vi "gfitsio-read-key-logical.vi"(7 "keyname":string, 8 "error in (no error)":errorcluster, 9 "default value":bool, 11 "gfits refnum":T1) -> (0 "error out":errorcluster, 1 "comment":string, 2 "value":bool, 3 "dup gfits refnum":T1)   [LabVIEW 2022 SP3, in "gfitsio.lvlib"]
doc: "Return the specified keyword. <B>default value</B> specifies the desired returned data type of the keyword value. Data type conversion will be performed for numeric values if the keyword value does not have the same data type. If the keyword does not exist or an error occurs <B>value</B> will be equal to <B>default value</B>."
uses:
  gfitsio.lvlib
  gfitsio-refnum.ctl
  cfitsio-datatypes.ctl
  gfitsio.dll
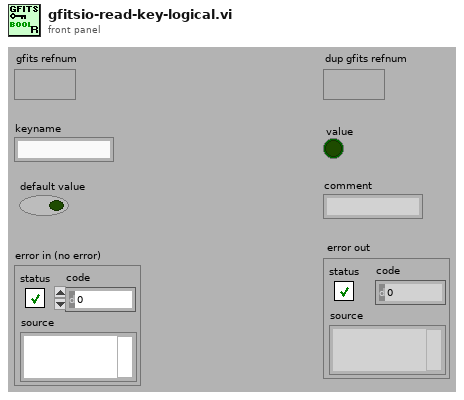
[diagram p1: front panel]
types:
  T1 = typedef "gfitsio.lvlib/gfitsio-refnum.ctl" = refnum<k1>
  T2 = typedef "gfitsio.lvlib/cfitsio-datatypes.ctl" = i32
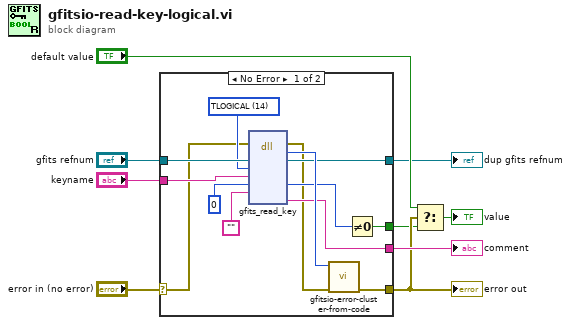
[diagram p0: block diagram]
diagram:
  n1 = case shown="No Error" "error in (no error)" {
    selector: "error in (no error)" -> [w11 w24]
    tunnel: [w21 w24] -> w3
    tunnel: "gfits refnum" -> [w19 w23]
    tunnel: [w20 w23] -> w1
    tunnel: "keyname" -> [w17 _]
    tunnel: [w12 _] -> w2
    tunnel: [w14 _] -> w4
    frame No Error {
      w18 = T2 14 items=["TBIT"=1, "TBYTE  (U8)"=11, "TSBYTE  (I8)"=12, "TLOGICAL"=14, "TSTRING"=16, "TUSHORT  (U16)"=20, "TSHORT  (I16)"=21, "TUINT"=31, "TULONG  (U32)"=40, "TLONG  (I32)"=41, "TFLOAT  (SGL)"=42, "TLONGLONG  (I64)"=81, "TDOUBLE  (DBL)"=82, "TCOMPLEX  (CSG)"=83, "TDOUBLECOMPLEX  (CDB)"=163] ("cfitsio datatype")
      n2 = dll-call lib="gfitsio.dll" fn="gfits_read_key"(error in=w11, "gfits refnum"=w19, "datatype"=w18, "keyname"=w17, "value"=u8 0, "units"="") -> (error out=w10:errorcluster, w22:i32, "gfits refnum"=w20:T1, "value"=w15:u8, "comment"=w14:string)  [unwired: 4 in, 3 out]
      n3 = call "gfitsio-error-cluster-from-code.vi"("error in (no error)"=w10, "error code"=w22) -> ("error out"=w21:errorcluster)  [unwired: 9 out]
      n4 = Not Equal To 0?(x=w15) -> (x != 0?=w12:bool)
    }
    frame Error {
    }
  }
  "error out" <- w3
  "dup gfits refnum" <- w1
  "comment" <- w4
  n5 = Select(t="default value", s=w3, f=w2) -> (s? t:f=→"value":bool)
